vi "Write Text to Output Directory.vi"(8 "error in (no error)":errorcluster, 11 "Parse Presentation in":refnum<class "Parse Presentation.lvclass">) -> (0 "error out":errorcluster, 3 "Parse Presentation out":refnum<class "Parse Presentation.lvclass">)   [LabVIEW 2015, in "Parse Presentation.lvclass"]
uses:
  Parse Presentation.lvclass
  Parse Presentation.lvclass/Parse Presentation.ctl
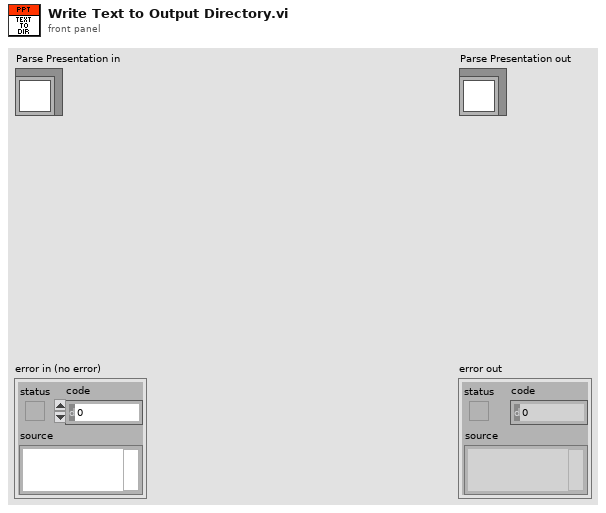
[diagram p1: front panel]
types:
  T1 = enum16{"open", "replace", "create", "open or create", "replace or create", "replace or create with confirmation"}
  T2 = typedef "Parse Presentation.lvclass/Slide Info..cluster.ctl" = cluster{"Slide":i32, "Text":string, "Images":string}
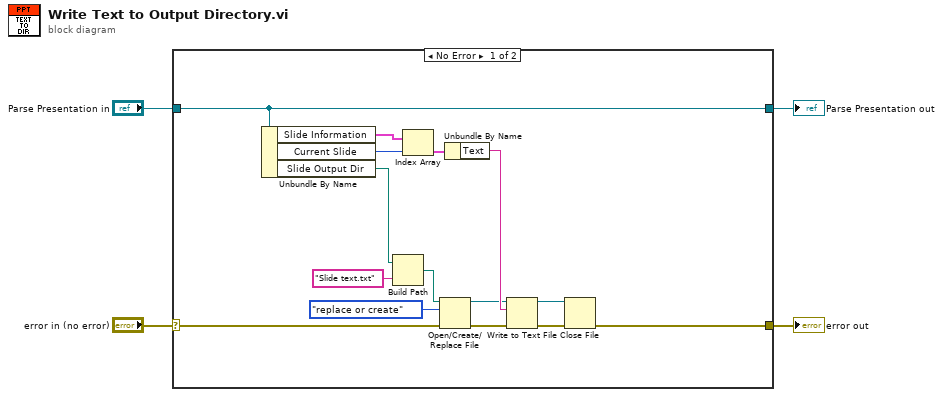
[diagram p0: block diagram]
diagram:
  n1 = case shown="No Error" "error in (no error)" {
    selector: "error in (no error)" -> [w7 w21]
    tunnel: [w6 w21] -> w3
    tunnel: [w11 w20] -> w1
    tunnel: "Parse Presentation in" -> [w11 w20]
    frame No Error {
      n2 = Unbundle By Name(w11) -> ("Slide Information"=w10:T2[], "Current Slide"=w9:i32, "Slide Output Dir"=w8:path)
      n3 = Build Path(base path=w8, name or relative path="Slide text.txt") -> (appended path=w17:path)
      n4 = Index Array(array=w10, index=w9) -> (element=w5:T2)
      n5 = Open/Create/Replace File(file path (use dialog)=w17, error in=w7, operation (0:open)=T1."replace or create") -> (refnum out=w15:refnum<file>, error out=w12:errorcluster)  [unwired: 3 in, 1 out]
      n6 = Unbundle By Name(w5) -> ("Text"=w16:string)
      n7 = Write to Text File(file (use dialog)=w15, text=w16, error in=w12) -> (refnum out=w19:refnum<file>, error out=w14:errorcluster)  [unwired: 1 in, 1 out]
      n8 = Close File(refnum=w19, error in=w14) -> (error out=w6:errorcluster)  [unwired: 1 out]
    }
    frame Error {
    }
  }
  "error out" <- w3
  "Parse Presentation out" <- w1
